vi "standard_analog_waveform_generator.vi"() -> ()   [LabVIEW 2025]
uses:
  <vilib>/measure/NI_MABase.lvlib
panel:
  in  "Number of Points":dbl=1000.0 format="%#_13g"
  in  "Sampling frequency":dbl=5000.0 format="%#_13g"
  in  "Together ON/OFF":bool
  out "Boolean":bool
  out "Boolean":bool
  in  "Output to DAQ":bool
  out "DAQ Output Voltage":waveform(dbl)[](graph)
  in  "Voltage Amplitude":i32=1
  in  "Frequency (Hz)":i32=10
  in  "Phase (degrees)":i32
  in  "Waveform":string(combo)="sine"
  in  "Phase (degrees)":i32
  in  "Waveform":string(combo)="sine"
  in  "Frequency (Hz)":i32=10
  in  "Voltage Amplitude":i32=1
  in  "stop":bool
  # "Waveform Generator (open-loop)"
  # "X-AXIS"
  # "Y-AXIS"
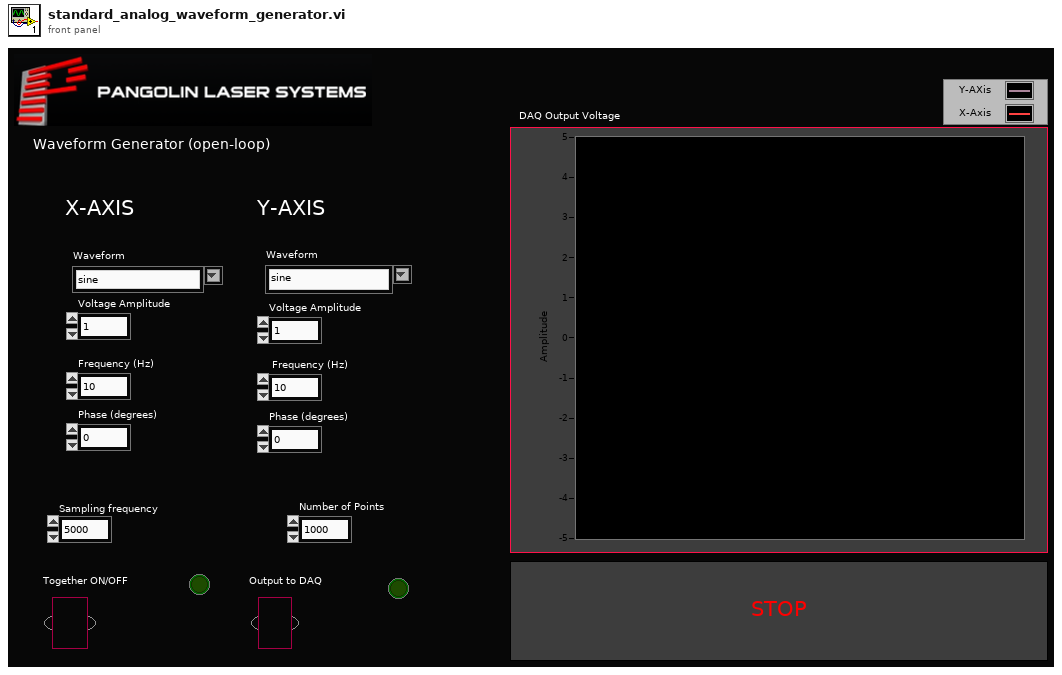
[diagram p1: front panel]
types:
  T1 = cluster{"Sampling frequency":dbl, "Number of Points":dbl}
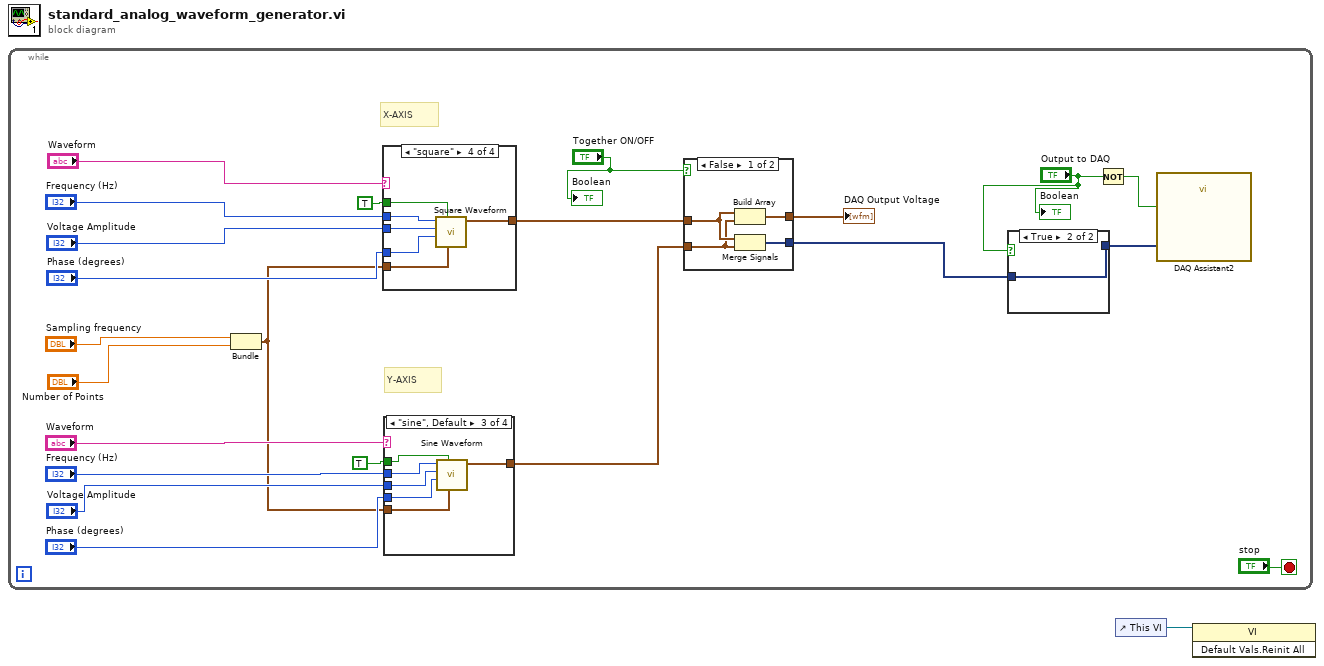
[diagram p0: block diagram]
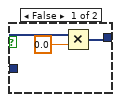
[diagram p2: hidden frame]
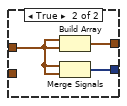
[diagram p3: hidden frame]
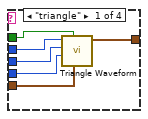
[diagram p4: hidden frame]
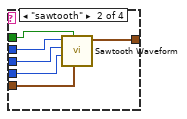
[diagram p5: hidden frame]
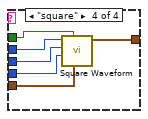
[diagram p6: hidden frame]
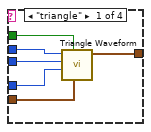
[diagram p7: hidden frame]
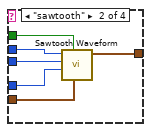
[diagram p8: hidden frame]
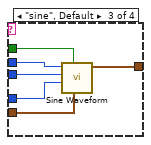
[diagram p9: hidden frame]
diagram:
  n1 = while {
    stop <- "stop" stop-if-true
    # "Y-AXIS"
    # "X-AXIS"
    n2 = Bundle("Sampling frequency"="Sampling frequency", "Number of Points"="Number of Points") -> (w7:T1)  [unwired: 1 in]
    n3 = case shown="\"square\"" "Waveform" {
      tunnel: "Voltage Amplitude" -> [w63 w69 w75 w82]
      tunnel: "Frequency (Hz)" -> [w64 w70 w76 w81]
      tunnel: w7 -> [w60 w66 w73 w80]
      tunnel: [w61 w65 w72 w79] -> w13
      tunnel: "Phase (degrees)" -> [w62 w68 w74 w78]
      tunnel: TRUE ("reset signal") -> [w59 w67 w71 w77]
      frame "triangle" {
        n4 = call <vilib>:"Triangle Waveform.vi"("sampling info"=w60, "reset signal"=w59, "phase"=w62, "amplitude"=w63, "frequency"=w64) -> ("signal out"=w61:waveform(dbl))  [unwired: 5 in, 1 out]
      }
      frame "sawtooth" {
        n5 = call <vilib>:"Sawtooth Waveform.vi"("sampling info"=w66, "reset signal"=w67, "phase"=w68, "amplitude"=w69, "frequency"=w70) -> ("signal out"=w65:waveform(dbl))  [unwired: 5 in, 1 out]
      }
      frame "sine", Default {
        n6 = call <vilib>:"Sine Waveform.vi"("sampling info"=w73, "reset signal"=w71, "phase"=w74, "amplitude"=w75, "frequency"=w76) -> ("signal out"=w72:waveform(dbl))  [unwired: 5 in, 1 out]
      }
      frame "square" {
        n7 = call <vilib>:"Square Waveform.vi"("sampling info"=w80, "reset signal"=w77, "phase"=w78, "amplitude"=w82, "frequency"=w81) -> ("signal out"=w79:waveform(dbl))  [unwired: 5 in, 1 out]
      }
    }
    n8 = case shown="\"sine\", Default" "Waveform" {
      tunnel: "Voltage Amplitude" -> [w38 w45 w50 w58]
      tunnel: "Frequency (Hz)" -> [w39 w46 w51 w57]
      tunnel: w7 -> [w35 w42 w48 w56]
      tunnel: [w36 w41 w47 w55] -> w12
      tunnel: TRUE ("reset signal") -> [w40 w43 w52 w54]
      tunnel: "Phase (degrees)" -> [w37 w44 w49 w53]
      frame "triangle" {
        n9 = call <vilib>:"Triangle Waveform.vi"("sampling info"=w35, "reset signal"=w40, "phase"=w37, "amplitude"=w38, "frequency"=w39) -> ("signal out"=w36:waveform(dbl))  [unwired: 5 in, 1 out]
      }
      frame "sawtooth" {
        n10 = call <vilib>:"Sawtooth Waveform.vi"("sampling info"=w42, "reset signal"=w43, "phase"=w44, "amplitude"=w45, "frequency"=w46) -> ("signal out"=w41:waveform(dbl))  [unwired: 5 in, 1 out]
      }
      frame "sine", Default {
        n11 = call <vilib>:"Sine Waveform.vi"("sampling info"=w48, "reset signal"=w52, "phase"=w49, "amplitude"=w50, "frequency"=w51) -> ("signal out"=w47:waveform(dbl))  [unwired: 5 in, 1 out]
      }
      frame "square" {
        n12 = call <vilib>:"Square Waveform.vi"("sampling info"=w56, "reset signal"=w54, "phase"=w53, "amplitude"=w58, "frequency"=w57) -> ("signal out"=w55:waveform(dbl))  [unwired: 5 in, 1 out]
      }
    }
    n13 = case shown="False" "Together ON/OFF" {
      tunnel: w13 -> [w31 w32]
      tunnel: w12 -> [w30 _]
      tunnel: [w29 w34] -> w2
      tunnel: [w28 w33] -> w11
      frame False {
        n14 = Build Array(w31, w30) -> (w28:waveform(dbl)[])
        n15 = Merge Signals(w31, w30) -> (w29:dynamicdata)
      }
      frame True {
        n16 = Build Array(w32, w32) -> (w33:waveform(dbl)[])
        n17 = Merge Signals(w32, w32) -> (w34:dynamicdata)
      }
    }
    "DAQ Output Voltage" <- w11
    n18 = case shown="True" "Output to DAQ" {
      tunnel: w2 -> [w24 w27]
      tunnel: [w25 w27] -> w3
      frame False {
        n19 = Multiply(x=w24, y=0.0) -> (x*y=w25:dynamicdata)
      }
      frame True {
      }
    }
    n20 = Not(x="Output to DAQ") -> (.not. x?=w5:bool)
    n21 = call "DAQ Assistant2"("data"=w3, "stop (F)"=w5) -> ()  [unwired: 15 in, 3 out]
    "Boolean" <- "Output to DAQ"
    "Boolean" <- "Together ON/OFF"
  }
  n22 = control-ref of="This VI"() -> (w1:refnum<vi>)
  n23 = invoke class="VI" method="Default Vals.Reinit All"(reference=w1) -> ()  [unwired: 2 in, 3 out]
